vi "Get_Plotted_Channel_Data.vi"(4 "Channel Names":string[](array[string])) -> (1 "Selected Data Cluster":cluster{"Selected Data":string[][]}[](array[cluster]))   [LabVIEW 2011]
uses:
  Results_plotter_Global.vi
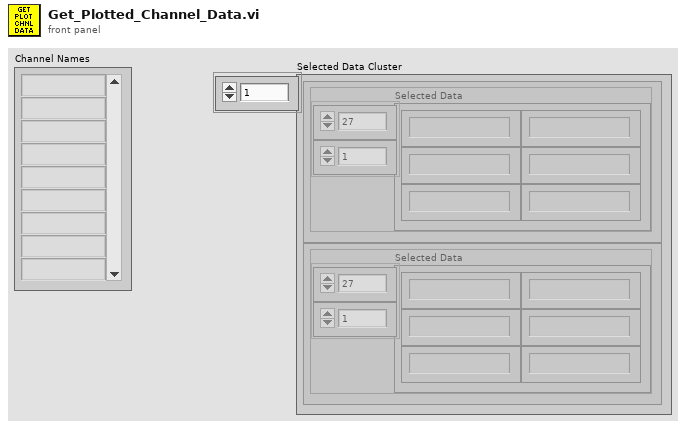
[diagram p1: front panel]
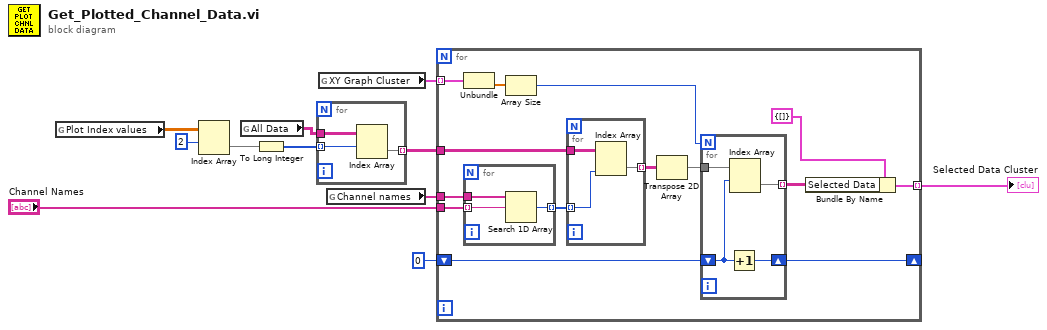
[diagram p0: block diagram]
diagram:
  n1 = global read "Results_plotter_Global.vi" "Plot Index values"() -> (w5:dbl[][])
  n2 = Index Array(array=w5, index (row)=2) -> (element=w8:dbl[])  [unwired: 1 in]
  n3 = global read "Results_plotter_Global.vi" "All Data"() -> (w6:string[][])
  n4 = To Long Integer(number=w8) -> (32bit integer=w7:i32[])
  n5 = for {
    tunnel: w7 -> [w14] mode=indexing
    tunnel: w6 -> [w13]
    tunnel: [w12] -> w4 mode=indexing
    n6 = Index Array(array=w13, index (row)=w14) -> (element=w12:string[])  [unwired: 1 in]
  }
  n7 = global read "Results_plotter_Global.vi" "XY Graph Cluster"() -> (w3:cluster{dbl[], dbl[]}[])
  n8 = global read "Results_plotter_Global.vi" "Channel names"() -> (w11:string[])
  n9 = for {
    tunnel: w11 -> [w28]
    tunnel: "Channel Names" -> [w27]
    tunnel: w4 -> [w24]
    tunnel: w3 -> [w23] mode=indexing
    tunnel: [w17] -> w2 mode=indexing
    shift-right: [w15] -> _
    shift-left: 0 ("size(s)") -> [w16]
    n10 = Unbundle(w23) -> (w26:dbl[])  [unwired: 1 out]
    n11 = for {
      tunnel: w28 -> [w36]
      tunnel: w27 -> [w38] mode=indexing
      tunnel: [w37] -> w25 mode=indexing
      n12 = Search 1D Array(1D array=w36, element=w38) -> (index of element=w37:i32)  [unwired: 1 in]
    }
    n13 = Array Size(array=w26) -> (size(s)=w20:i32)
    n14 = for {
      tunnel: w25 -> [w34] mode=indexing
      tunnel: w24 -> [w35]
      tunnel: [w33] -> w22 mode=indexing
      n15 = Index Array(array=w35, index (col)=w34) -> (element=w33:string[])  [unwired: 1 in]
    }
    n16 = Transpose 2D Array(2D array=w22) -> (transposed array=w21:string[][])
    n17 = for {
      N: w20 -> [_]
      tunnel: w21 -> [w32]
      tunnel: [w31] -> w18 mode=indexing
      shift-right: [w29] -> w15
      shift-left: w16 -> [w30]
      n18 = Increment(x=w30) -> (x+1=w29:i32)
      n19 = Index Array(array=w32, index (row)=w30) -> (element=w31:string[])  [unwired: 1 in]
    }
    n20 = Bundle By Name(cluster=cluster{"Selected Data":string[][]} {"Selected Data"=[]} ("Data"), "Selected Data"=w18) -> (w17:cluster{"Selected Data":string[][]})
  }
  "Selected Data Cluster" <- w2
